vi "test Find Disabled Custom Devices.vi"(8 "error in":errorcluster, 11 "TestCase in":refnum<class "Scripting.lvclass">) -> (0 "error out":errorcluster, 3 "TestCase out":refnum<class "Scripting.lvclass">)   [LabVIEW 2020, in "Scripting.lvclass"]
uses:
  Scripting.lvclass
  Scripting.lvclass/Scripting.ctl
  Scripting/Ballard/Ballard ARINC 429 Scripting.lvlib
  <vilib>/addons/_JKI Toolkits/VI Tester/TestCase.llb/TestCase.lvclass
  C:/Program Files (x86)/National Instruments/LabVIEW 2020/vi.lib/addons/_JKI Toolkits/VI Tester/TestCase.llb/TestCase.lvclass
  C:/dev/git/niveristand-ballard-arinc429-custom-device/Source/Custom Device Support/Tests/Unit/Scripting/Scripting.lvclass
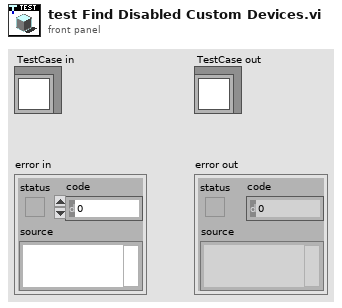
[diagram p1: front panel]
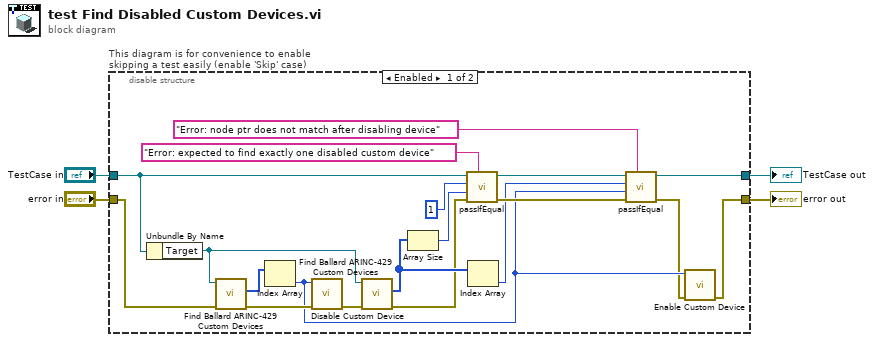
[diagram p0: block diagram]
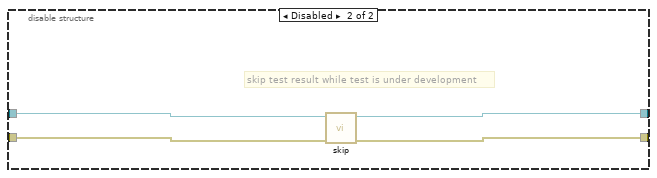
[diagram p2: hidden frame]
diagram:
  n1 = disable-structure "This diagram is for convenience to enable skipping a test easily (enable 'Skip' case)" shown="Enabled" {
    disable-tunnel: "TestCase in" -> [w18 w27]
    disable-tunnel: [w11 w25] -> w4
    disable-tunnel: [w6 w26] -> w2
    disable-tunnel: "error in" -> [w23 w24]
    frame Enabled {
      n2 = Unbundle By Name(w18) -> ("Target"=w16:refnum<k24>)
      n3 = call "Find Ballard ARINC-429 Custom Devices.vi"("error in"=w23, "target in"=w16) -> ("error out"=w20:errorcluster, "Ballard ARINC 429 custom devices"=w21:u64[])  [unwired: 7 in, 1 out]
      n4 = Index Array(array=w21) -> (element=w8:u64)  [unwired: 1 in]
      n5 = call "Disable Custom Device.vi"("error in (no error)"=w20, "Ballard ARINC 429 ref"=w8) -> ("error out"=w17:errorcluster)  [unwired: 8 in, 1 out]
      n6 = call "Find Ballard ARINC-429 Custom Devices.vi"("error in"=w17, "target in"=w16) -> ("error out"=w7:errorcluster, "Ballard ARINC 429 custom devices"=w13:u64[])  [unwired: 7 in, 1 out]
      n7 = Array Size(array=w13) -> (size(s)=w14:i32)
      n8 = call-dynamic "passIfEqual.vi"("custom report message (\"\")"="Error: expected to find exactly one disabled custom device" ("custom report message (\"\")"), "error in (no error)"=w7, "y"=w14, "x"=1, "TestCase in"=w18) -> ("error out"=w22:errorcluster, "TestCase out"=w12:refnum<class "Scripting.lvclass">)  [unwired: 5 in]
      n9 = Index Array(array=w13) -> (element=w10:u64)  [unwired: 1 in]
      n10 = call-dynamic "passIfEqual.vi"("custom report message (\"\")"="Error: node ptr does not match after disabling device" ("custom report message (\"\")"), "error in (no error)"=w22, "y"=w8, "x"=w10, "TestCase in"=w12) -> ("error out"=w5:errorcluster, "TestCase out"=w11:refnum<class "Scripting.lvclass">)  [unwired: 5 in]
      n11 = call "Enable Custom Device.vi"("error in (no error)"=w5, "Ballard ARINC 429 ref"=w8) -> ("error out"=w6:errorcluster)  [unwired: 8 in, 1 out]
    }
    frame Disabled {
      # "skip test result while test is under development"
      n12 = call <vilib>:"skip.vi"("error in (no error)"=w24, "TestCase in"=w27) -> ("error out"=w26:errorcluster, "TestCase out"=w25:refnum<class "Scripting.lvclass">)  [unwired: 8 in]
    }
  }
  "error out" <- w2
  "TestCase out" <- w4
